vi "lee-eeprom.vi"(0 "Equipo Nº":u8, 3 "COM DATA":T1) -> (2 "fallo final":bool, 4 "COM FAIL":bool caption="COM\nFAIL", 5 "LECTURA":string, 6 "error out":errorcluster)   [LabVIEW 2010]
panel:
  in  "Err+":u8
  out "comando":string
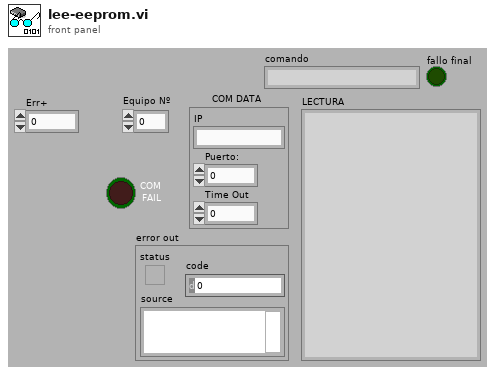
[diagram p1: front panel]
types:
  T1 = cluster{"IP ":string, "Puerto:":u16, "Time Out":u16}
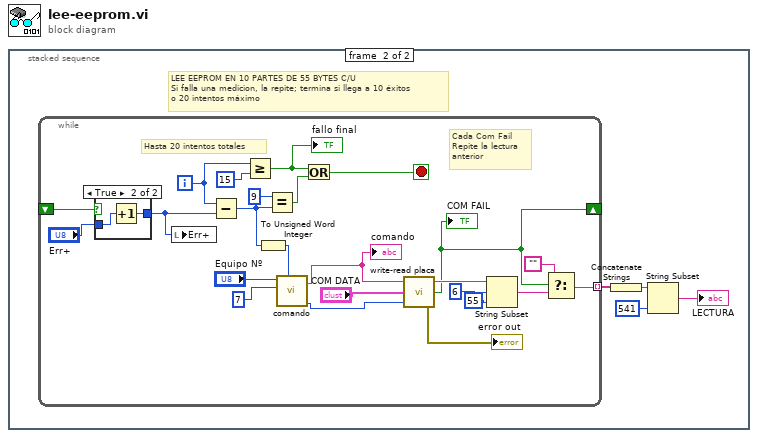
[diagram p0: block diagram]
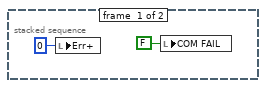
[diagram p2: hidden frame]
diagram:
  n1 = stacked-sequence {
    frame #0 {
      n2 = local write "Err+"(u8 0 ("Err+")) -> ()
      n3 = local write "COM FAIL"(FALSE ("COM FAIL")) -> ()
    }
    frame #1 {
      # "LEE EEPROM EN 10 PARTES DE 55 BYTES C/U\nSi falla una medicion, la repite; termina si llega a 10 éxitos\no 20 intentos máximo"
      n4 = while {
        tunnel: [w10] -> w6 mode=indexing
        shift-right: [w9] -> _
        shift-left: _ -> [w14]
        i -> [w17]
        stop <- w12 stop-if-true
        # "Hasta 20 intentos totales"
        # "Cada Com Fail\nRepite la lectura\nanterior"
        n5 = case shown="True" w14 {
          tunnel: "Err+" -> [w31 w33]
          tunnel: [w31 w32] -> w7
          frame False {
          }
          frame True {
            n6 = Increment(x=w33) -> (x+1=w32:u8)
          }
        }
        n7 = local write "Err+"(w7) -> ()
        n8 = Subtract(x=w17, y=w7) -> (x-y=w19:i32)
        n9 = Greater Or Equal?(x=w17, y=15) -> (x >= y?=w16:bool)
        "fallo final" <- w16
        n10 = To Unsigned Word Integer(number=w19) -> (unsigned 16bit integer=w21:u16)
        n11 = Equal?(x=9, y=w19) -> (x = y?=w18:bool)
        n12 = call "comando.vi"("BYTES IN"=w21, "Comando:"=u8 7, "Equipo Nº"="Equipo Nº") -> ("Bytes OUT"=w24:u16, "comando"=w25:string)  [unwired: 4 in]
        "comando" <- w25
        n13 = Or(x=w16, y=w18) -> (x .or. y?=w12:bool)
        n14 = call "write-read placa.vi"("Write Command"=w25, "COM DATA"="COM DATA", "bytes"=w24) -> ("LECTURA"=w28:string, "COM FAIL"=w9:bool, "error out"=→"error out":errorcluster)  [unwired: 2 in]
        "COM FAIL" <- w9
        n15 = String Subset(string=w28, offset (0)=6, length (rest)=55 ("offset (0)")) -> (substring=w11:string)
        n16 = Select(t="", s=w9, f=w11) -> (s? t:f=w10:string)
      }
      n17 = Concatenate Strings(w6) -> (w3:string)
      n18 = String Subset(string=w3, length (rest)=541 ("offset (0)")) -> (substring=→"LECTURA":string)  [unwired: 1 in]
    }
  }
